vi "Unpack for gRPC.vi"(8 "error in":errorcluster, 9 "configuration / results":enum16{"Configuration", "Results"}(ring), 10 "any":T1, 11 "measurement customizations in":refnum<class "Measurement Plugin.lvclass">) -> (0 "error out":errorcluster, 2 "data value":variant, 3 "measurement customizations out":refnum<class "Measurement Plugin.lvclass">)   [LabVIEW 2022 SP3, in "Single Tone - Digital Mic.lvlib" / "Measurement Plugin.lvclass"]
uses:
  Measurement Plugin.lvclass
  <vilib>/gRPC/LabVIEW gRPC Library/Shared/Any.ctl
  C:/Program Files/National Instruments/LabVIEW 2022/vi.lib/Plug-In SDKs/Measurements/Measurement Plugin Service/Measurement Plugin Service.lvclass
  Measurement Configuration.ctl
  shared/measurements/controls/lowpass filter.ctl
  shared/measurements/controls/weighting filter.ctl
  shared/measurements/controls/highpass filter.ctl
  shared/measurements/controls/measurement units.ctl
  Measurement Results.ctl
  a521b266-ce99-437c-923d-067dcf1e07fd.vi
  3ecd018e-d556-4cbc-bc60-c4ba57204520.vi
  <vilib>/gRPC/LabVIEW gRPC Library/Server API/Translate Protobuf Error.vi
  <vilib>/AdvancedString/1D String Array to Delimited String.vi
  <vilib>/gRPC/LabVIEW gRPC Library/Server API/Server/Get Server DLL Path.vi
  Single Tone - Digital Mic.lvlib
  <vilib>/Plug-In SDKs/Measurements/Measurement Plugin Service/Measurement Plugin Service.lvclass
  <vilib>/gRPC/LabVIEW gRPC Library/grpc-lvsupport-release.lvlib
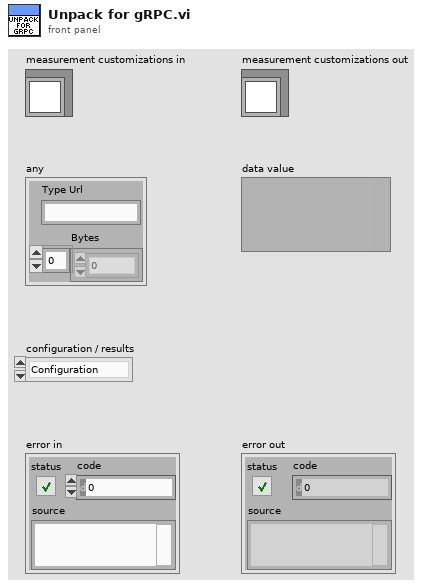
[diagram p1: front panel]
types:
  T1 = typedef "grpc-lvsupport-release.lvlib/Any.ctl" = cluster{"Type Url":string, "Bytes":u8[]}
  T2 = typedef "grpc-lvsupport-release.lvlib/grpcId.ctl" = u64
  T3 = typedef "Single Tone - Digital Mic.lvlib/Measurement Configuration.ctl" = cluster{"digital channel list":string, "input cfg file":string, "digital mic sensitivity (dBFS)":dbl, "ref mic channel":string, "ref mic sensitivity (mV/Pa)":dbl, "output channel":string, "signal frequency":dbl, "output level (dBSPL)":dbl, "output voltage ratio":dbl, "lowpass filter":T4, "weighting filter":T5, "highpass filter":T6, "band start":dbl, "band stop":dbl, "min measurement cycles":u32, "min measurement time (s)":dbl, "min settling cycles":u32, "min settling time (s)":dbl, "SNR units":T7, "THD+N units":T7, "THD units":T7}
  T4 = typedef "lowpass filter.ctl" = enum32{"No filter", "AES17 20kHz", "AES17 40kHz"}
  T5 = typedef "weighting filter.ctl" = enum32{"Linear", "A-weighting", "B-weighting", "C-weighting"}
  T6 = typedef "highpass filter.ctl" = enum32{"DC", "AC"}
  T7 = typedef "measurement units.ctl" = enum32{"dB", "%", "x/y"}
  T8 = typedef "Single Tone - Digital Mic.lvlib/Measurement Results.ctl" = cluster{"channel name":string, "frequency (Hz)":dbl, "amplitude (Pa RMS)":dbl, "amplitude (dBSPL)":dbl, "microphone sensitivity (dBFS)":dbl, "SNR":dbl, "THD+N":dbl, "THD":dbl, "wfm - dt":dbl, "wfm - data":dbl[], "fft - f0":dbl, "fft - df":dbl, "fft - data":dbl[], "ref mic wfm - dt":dbl, "ref mic wfm - data":dbl[]}
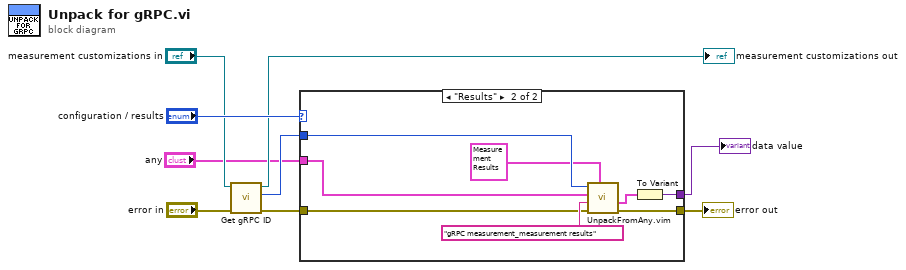
[diagram p0: block diagram]
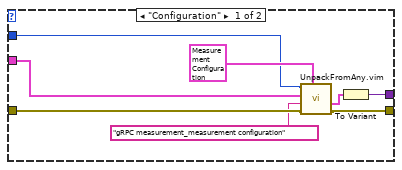
[diagram p2: hidden frame]
diagram:
  n1 = call <vilib>:"Get gRPC ID.vi"("error in"="error in", "measurement plugin service in"="measurement customizations in") -> ("error out"=w6:errorcluster, "gRPC ID"=w3:T2, "measurement plugin service out"=→"measurement customizations out":refnum<class "Measurement Plugin.lvclass">)  [unwired: 7 in]
  n2 = case shown="\"Results\"" "configuration / results" {
    tunnel: w6 -> [w15 w19]
    tunnel: "any" -> [w10 w18]
    tunnel: w3 -> [w12 w22]
    tunnel: [w16 w23] -> w9
    tunnel: [w17 w25] -> w1
    frame "Configuration" {
      n3 = call "UnpackFromAny.vim"("Data Type"=T3 {"digital channel list"="Lorem ipsum dolor sit", "input cfg file"="", "digital mic sensitivity (dBFS)"=1.2, "ref mic channel"="7821\\PCMo 0", "ref mic sensitivity (mV/Pa)"=32.0, "output channel"="7821\\PCMo 0", "signal frequency"=-32.0, "output level (dBSPL)"=1.0, "output voltage ratio"=1.0, "lowpass filter"=enum."No filter", "weighting filter"=enum."Linear", "highpass filter"=enum."DC", "band start"=20.0, "band stop"=20000.0, "min measurement cycles"=20, "min measurement time (s)"=0.1, "min settling cycles"=0, "min settling time (s)"=0.0, "SNR units"=enum."dB", "THD+N units"=enum."dB", "THD units"=enum."dB"} ("Measurement Configuration"), "error in"=w15, "Message Type"="gRPC measurement_measurement configuration", "Any"=w10, "gRPCid in"=w12) -> ("error out"=w16:errorcluster, "Unpacked Value"=w14:T3)  [unwired: 4 in, 1 out]
      n4 = To Variant(anything=w14) -> (Variant=w17:variant)
    }
    frame "Results" {
      n5 = call "UnpackFromAny.vim"("Data Type"=T8 {"channel name"="Empty", "frequency (Hz)"=0.0, "amplitude (Pa RMS)"=0.0, "amplitude (dBSPL)"=0.0, "microphone sensitivity (dBFS)"=0.0, "SNR"=0.0, "THD+N"=0.0, "THD"=0.0, "wfm - dt"=0.0, "wfm - data"=[], "fft - f0"=0.0, "fft - df"=0.0, "fft - data"=[], "ref mic wfm - dt"=0.0, "ref mic wfm - data"=[]} ("Measurement Results"), "error in"=w19, "Message Type"="gRPC measurement_measurement results", "Any"=w18, "gRPCid in"=w22) -> ("error out"=w23:errorcluster, "Unpacked Value"=w24:T8)  [unwired: 4 in, 1 out]
      n6 = To Variant(anything=w24) -> (Variant=w25:variant)
    }
  }
  "error out" <- w9
  "data value" <- w1
